vi "CryoServer Initialize.vi"(8 "error in (no error)":errorcluster, 9 "Show GUI? (False)":bool, 10 "address":string, 11 "CryoServer in":refnum<class "CryoServer.lvclass">) -> (0 "error out":errorcluster, 3 "CryoServer out":refnum<class "CryoServer.lvclass">)   [LabVIEW 2021, in "CryoServer.lvclass"]
uses:
  CryoServer.lvclass
  CryoServer.lvclass/CryoServer.ctl
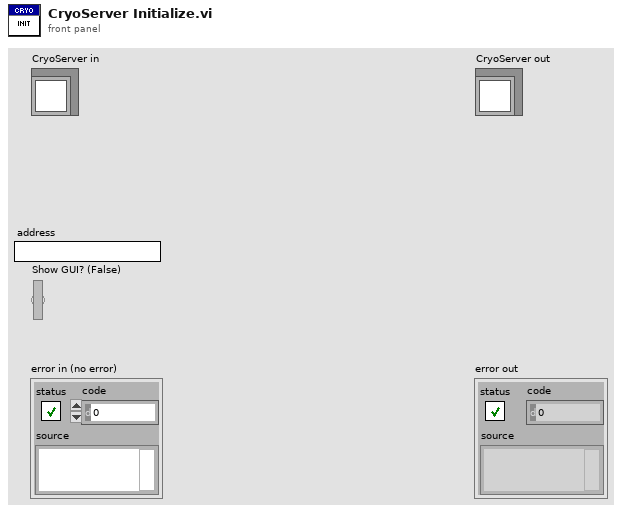
[diagram p1: front panel]
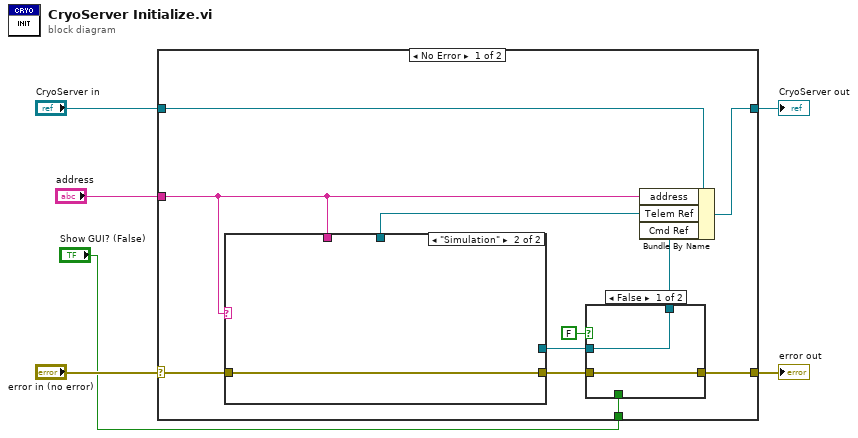
[diagram p0: block diagram]
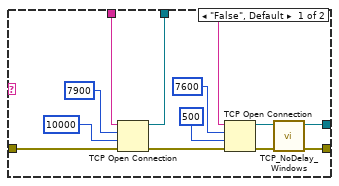
[diagram p2: hidden frame]
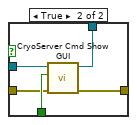
[diagram p3: hidden frame]
diagram:
  n1 = case shown="No Error" "error in (no error)" {
    selector: "error in (no error)" -> [w17 w39]
    tunnel: [w9 w39] -> w5
    tunnel: [w15 w38] -> w3
    tunnel: "CryoServer in" -> [w14 w38]
    tunnel: "address" -> [w7 _]
    tunnel: "Show GUI? (False)" -> [w13 _]
    frame No Error {
      n2 = case shown="\"Simulation\"" w7 {
        tunnel: w17 -> [w29 w30]
        tunnel: w7 -> [w23 _]
        tunnel: [w22 _] -> w16
        tunnel: [w19 _] -> w12
        tunnel: [w18 w30] -> w11
        frame "False", Default {
          n3 = TCP Open Connection(address=w23, remote port or service name=u16 7900, timeout ms (60000)=10000, error in (no error)=w29) -> (connection ID=w22:refnum<k5>, error out=w26:errorcluster)  [unwired: 1 in]
          n4 = TCP Open Connection(address=w23, remote port or service name=u16 7600, timeout ms (60000)=500, error in (no error)=w26) -> (connection ID=w21:refnum<k5>, error out=w20:errorcluster)  [unwired: 1 in]
          n5 = call "TCP_NoDelay_Windows.vi"("error in (no error)"=w20, "connID"=w21) -> ("error out"=w18:errorcluster, "connID 2"=w19:refnum<k5>)  [unwired: 4 in]
        }
        frame "Simulation" {
        }
      }
      n6 = case shown="False" FALSE {
        tunnel: w13 -> [_ w37]
        tunnel: w12 -> [w32 w36]
        tunnel: w11 -> [w31 w35]
        tunnel: [w32 w34] -> w10
        tunnel: [w31 w33] -> w9
        frame False {
        }
        frame True {
          n7 = call "CryoServer Cmd Show GUI.vi"("error in (no error)"=w35, "Show GUI? (False)"=w37, "connection ID"=w36) -> ("error out"=w33:errorcluster, "connection ID out"=w34:refnum<k5>)  [unwired: 7 in]
        }
      }
      n8 = Bundle By Name(cluster=w14, "address"=w7, "Telem Ref"=w16, "Cmd Ref"=w10) -> (w15:refnum<class "CryoServer.lvclass">)
    }
    frame Error {
    }
  }
  "error out" <- w5
  "CryoServer out" <- w3
